vi "Get Category.vi"(8 "error in (no error)":errorcluster, 11 "CVT editor node in":refnum<class "CVT editor node.lvclass">) -> (0 "error out":errorcluster, 2 "Category":string, 3 "CVT editor node out":refnum<class "CVT editor node.lvclass">)   [LabVIEW 2013, in "CVT editor node.lvclass"]
uses:
  CVT editor node.lvclass
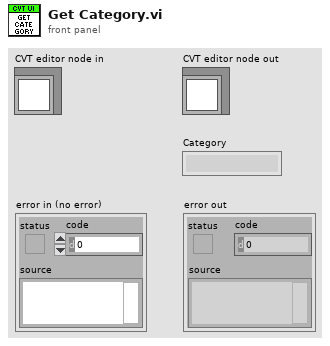
[diagram p1: front panel]
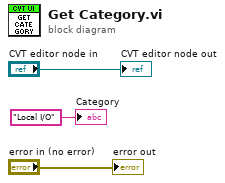
[diagram p0: block diagram]
diagram:
  "error out" <- "error in (no error)"
  "CVT editor node out" <- "CVT editor node in"
  "Category" <- "Local I/O" ("Category")
